vi "ExSubNframeColMultiImageFast.vi"(2 "image handles":u32[](array[numeric]), 3 "error in (no error)":errorcluster, 4 "Number of Images":u32=1 min=1 step=1, 5 "Handle Cluster":T1) -> (0 "error out":errorcluster, 1 "Handle Cluster":T1)   [LabVIEW 2010]
panel:
  # "ExSubNframeCol:\nThis is a sub VI that collects N frames from the camera\nsystem. This assumes camera has been setup and \ninitialized and that the start camera is done. It also \nassumes the camera has circular buffer capabillities.\nThis is not true for all cameras, especially older \nPhotometrics cameras."
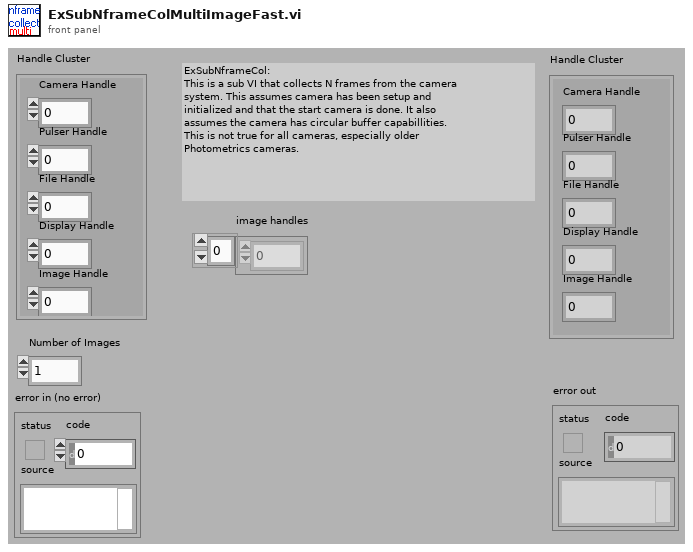
[diagram p1: front panel]
types:
  T1 = cluster{"Camera Handle":u32, "Pulser Handle":u32, "File Handle":u32, "Display Handle":u32, "Image Handle":u32}
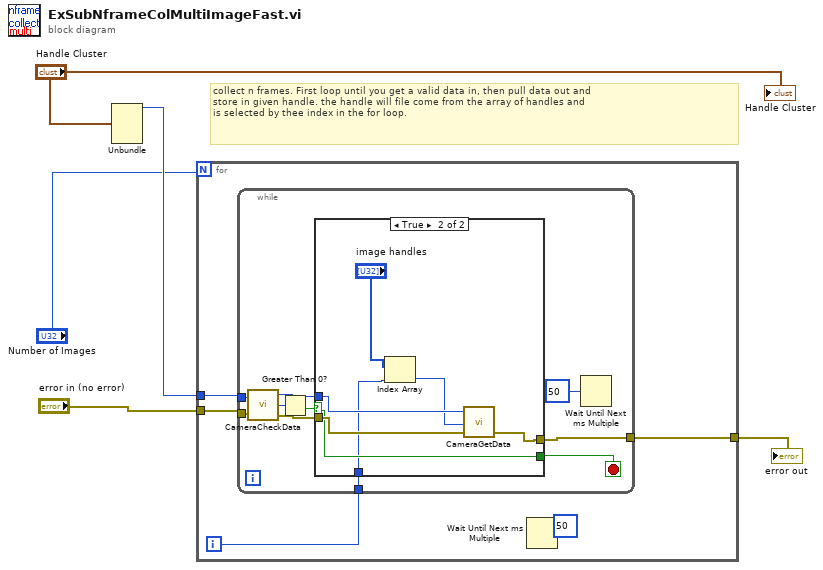
[diagram p0: block diagram]
diagram:
  # "collect n frames. First loop until you get a valid data in, then pull data out and \nstore in given handle. the handle will file come from the array of handles and\nis selected by thee index in the for loop."
  n1 = Unbundle("Handle Cluster") -> ("Camera Handle"=w5:u32)  [unwired: 4 out]
  n2 = for {
    N: "Number of Images" -> [_]
    tunnel: w5 -> [w10]
    tunnel: "error in (no error)" -> [w9]
    tunnel: [w6] -> w1
    i -> [w7]
    n3 = while {
      tunnel: w9 -> [w19]
      tunnel: w10 -> [w18]
      tunnel: [w13] -> w6
      tunnel: w7 -> [w11]
      stop <- w14 stop-if-true
      n4 = call <userlib>:"CameraCheckData.vi"("Camera Handle"=w18, "error in"=w19) -> ("Camera Handle"=w16:u32, "Number Of Frames Available"=w20:i32, "error out"=w15:errorcluster)
      n5 = Greater Than 0?(x=w20) -> (x > 0?=w17:bool)
      n6 = case shown="True" w17 {
        selector: w17 -> [w21 w27]
        tunnel: w16 -> [_ w29]
        tunnel: w15 -> [w22 w28]
        tunnel: [w21 w27] -> w14
        tunnel: [w22 w26] -> w13
        tunnel: w11 -> [_ w25]
        frame False {
        }
        frame True {
          n7 = Index Array(array="image handles", index=w25) -> (element=w23:u32)
          n8 = call <userlib>:"CameraGetData.vi"("error in"=w28, "Data Handle"=w23, "Camera Handle"=w29) -> ("error out"=w26:errorcluster)  [unwired: 2 out]
        }
      }
      n9 = Wait Until Next ms Multiple(millisecond multiple=u32 50) -> ()  [unwired: 1 out]
    }
    n10 = Wait Until Next ms Multiple(millisecond multiple=u32 50) -> ()  [unwired: 1 out]
  }
  "error out" <- w1
  "Handle Cluster" <- "Handle Cluster"
